vi "sort wheel table.vi"(7 "Wheel table":string[][](array[string]), 11 "error in (no error)":errorcluster) -> (8 "Paged groups":string[][][](array[string]), 15 "error out":errorcluster)   [LabVIEW 2016]
doc: "This vi takes a wheel list and sorts it into a sereis of groups to be run. It creates a 3d array where each page is a group(0-6, plus blanks and qa= page 7). Each row of each page is the information of 1 sample"
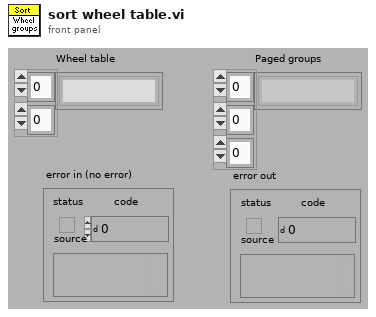
[diagram p1: front panel]
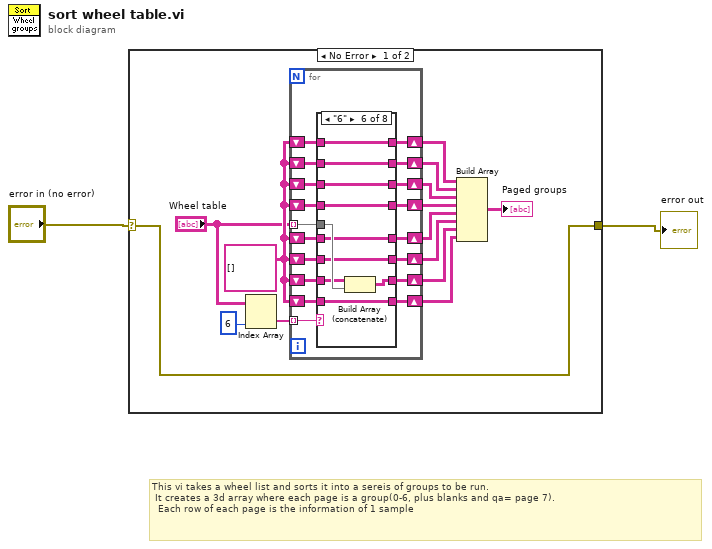
[diagram p0: block diagram]
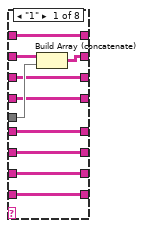
[diagram p2: hidden frame]
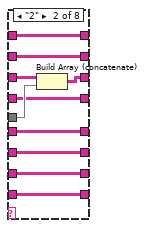
[diagram p3: hidden frame]
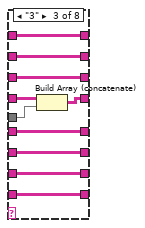
[diagram p4: hidden frame]
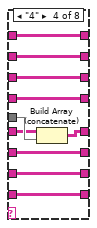
[diagram p5: hidden frame]
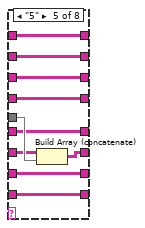
[diagram p6: hidden frame]
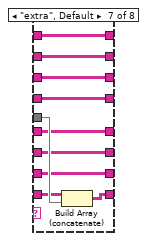
[diagram p7: hidden frame]
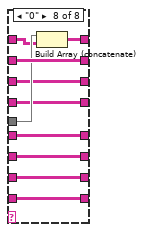
[diagram p8: hidden frame]
diagram:
  # "This vi takes a wheel list and sorts it into a sereis of groups to be run.\n It creates a 3d array where each page is a group(0-6, plus blanks and qa= page 7).\n  Each row of each page is the information of 1 sample"
  n1 = case shown="No Error" "error in (no error)" {
    selector: "error in (no error)" -> [w3 w115]
    tunnel: [w3 w115] -> w1
    frame No Error {
      w7 = string[][] []
      n2 = Index Array(array="Wheel table", index (col)=6 ("disabled index (col)")) -> (element=w6:string[])  [unwired: 1 in]
      n3 = for {
        tunnel: "Wheel table" -> [w33] mode=indexing
        tunnel: w6 -> [w34] mode=indexing
        shift-right: [w32] -> w8
        shift-left: w7 -> [w31]
        shift-right: [w30] -> w9
        shift-left: w7 -> [w29]
        shift-right: [w28] -> w10
        shift-left: w7 -> [w27]
        shift-right: [w26] -> w11
        shift-left: w7 -> [w25]
        shift-right: [w24] -> w12
        shift-left: w7 -> [w23]
        shift-right: [w22] -> w13
        shift-left: w7 -> [w21]
        shift-right: [w20] -> w14
        shift-left: w7 -> [w19]
        shift-right: [w18] -> w15
        shift-left: w7 -> [w17]
        n4 = case shown="\"6\"" w34 {
          tunnel: w33 -> [w43 w53 w63 w73 w83 w93 w103 w113]
          tunnel: [w44 w54 w64 w74 w84 w94 w104 w111] -> w32
          tunnel: w31 -> [w44 w54 w64 w74 w84 w94 w104 w112]
          tunnel: [w41 w52 w62 w72 w82 w92 w102 w114] -> w30
          tunnel: w29 -> [w42 w52 w62 w72 w82 w92 w102 w114]
          tunnel: [w40 w51 w61 w71 w81 w91 w101 w110] -> w28
          tunnel: w27 -> [w40 w50 w61 w71 w81 w91 w101 w110]
          tunnel: [w39 w49 w60 w70 w80 w90 w100 w109] -> w26
          tunnel: w25 -> [w39 w49 w59 w70 w80 w90 w100 w109]
          tunnel: [w38 w48 w58 w69 w79 w89 w99 w108] -> w24
          tunnel: w23 -> [w38 w48 w58 w68 w79 w89 w99 w108]
          tunnel: [w37 w47 w57 w67 w78 w88 w98 w107] -> w22
          tunnel: w21 -> [w37 w47 w57 w67 w77 w88 w98 w107]
          tunnel: [w36 w46 w56 w66 w76 w87 w95 w106] -> w20
          tunnel: w19 -> [w36 w46 w56 w66 w76 w86 w95 w106]
          tunnel: [w35 w45 w55 w65 w75 w85 w97 w105] -> w18
          tunnel: w17 -> [w35 w45 w55 w65 w75 w85 w96 w105]
          frame "1" {
            n5 = Build Array (concatenate)(w42, w43) -> (w41:string[][])
          }
          frame "2" {
            n6 = Build Array (concatenate)(w50, w53) -> (w51:string[][])
          }
          frame "3" {
            n7 = Build Array (concatenate)(w59, w63) -> (w60:string[][])
          }
          frame "4" {
            n8 = Build Array (concatenate)(w68, w73) -> (w69:string[][])
          }
          frame "5" {
            n9 = Build Array (concatenate)(w77, w83) -> (w78:string[][])
          }
          frame "6" {
            n10 = Build Array (concatenate)(w86, w93) -> (w87:string[][])
          }
          frame "extra", Default {
            n11 = Build Array (concatenate)(w96, w103) -> (w97:string[][])
          }
          frame "0" {
            n12 = Build Array (concatenate)(w113, w112) -> (w111:string[][])
          }
        }
      }
      n13 = Build Array(w8, w9, w10, w11, w12, w13, w14, w15) -> (→"Paged groups":string[][][])
    }
    frame Error {
    }
  }
  "error out" <- w1
